vi "SVT Coherent Output Power Subset.vi"(0 "scaled signal X [EUx]":waveform(dbl)={"t0"=timestamp(0 s since 1904-01-01), "dt"=1e-05, "Y"=[]}, 1 "scaled signal Y [EUy]":waveform(dbl)={"t0"=timestamp(0 s since 1904-01-01), "dt"=1e-05, "Y"=[]}, 2 "window":T10=1 items=["None"=0, "Hanning"=1, "Hamming"=2, "Blackman-Harris"=3, "Exact Blackman"=4, "Blackman"=5, "Flat Top"=6, "4 Term B-Harris "=7, "7 Term B-Harris"=8, "Low Sidelobe"=9, "Force - Exponential"=10, "Blackman Nuttall"=11, "Triangle"=30, "Bartlett-Hanning"=31, "Bohman"=32, "Parzen"=33, "Welch"=34, "Kaiser"=60, "Dolph-Chebyshev"=61, "Gaussian"=62], 3 "frequency range":T7={"start frequency"=1000.0, "stop frequency"=5000.0} {"stop frequency" min=0.0 format="%.2f"; "start frequency" min=0.0 format="%.2f"}, 4 "dB On (T)":bool=TRUE, 5 "error in (no error)":errorcluster, 7 "averaging parameters":T8={"averaging mode"=enum."No averaging", "weighting mode"=enum."Exponential", "number of averages"=10, "linear mode"=enum."One shot"}, 8 "force/exp settings":T9={"force window [%]"=50.0, "exp window [%]"=10.0} {"exp window [%]" min=0.0 max=100.0 format="%.2f"; "force window [%]" min=0.0 max=100.0 format="%.2f"}, 9 "restart averaging (F)":bool) -> (11 "averaging done":bool, 12 "coherence":cluster{"f0":dbl, "df":dbl, "coherence":dbl[]}={"f0"=nan, "df"=inf, "coherence"=[]} {"coherence" format="%.2p"; "df" format="%.2p"; "f0" format="%.2p"}, 13 "averages completed":dbl, 14 "coherent output power [dB EUy]":cluster{"f0":dbl, "df":dbl, "magnitude":dbl[]}={"f0"=nan, "df"=inf, "magnitude"=[]} {"magnitude" format="%.2p"; "df" format="%.2p"; "f0" format="%.2p"}, 15 "unit label":string, 18 "spectrum info":T1={"channel name"="", "description"="", "x-axis units"=1, "spectral info"={"spectrum type"=enum."Power [Magnitude^2]", "linear/dB"=enum."linear", "window"=0, "window size"=0, "FFT size"=0}, "engineering units"=0, "custom label"="", "dB reference [EU]"=0.0, "peak units"=enum."rms", "weighting filter"=0, "spectral density?"=FALSE, "unit label"="", "spectrum skewed?"=FALSE, "complimentary spectrum units"=enum."none"} {"x-axis units" items=["Time (s)"=0, "Frequency-CB (Hz)"=1, "Frequency-CPB (Hz)"=1248, "Frequency-Arbitrary (Hz)"=2357, "Quefrency (s)"=2, "Revolutions (rev)"=3, "Order"=4, "Speed (RPM)"=11, "Speed (rad/s)"=21, "Index"=65535]; "weighting filter" items=["Linear", "A-weighting", "B-weighting", "C-weighting", "ITU-R 468-4", "Dolby", "CCITT", "C-message", "Wb", "Wc", "Wd", "We", "Wf", "Wh", "Wj", "Wk", "Wm", "AES17 20 kHz lowpass", "AES17 40 kHz lowpass", "AES17 20 kHz highpass", "AES17 40 kHz highpass"]; "dB reference [EU]" format="%.2f"; "engineering units" items=["custom..."=0, "V"=1, "A"=21, "C"=30, "pC"=31, "s"=32, "-"=29, "Pa"=2, "N"=20, "g"=3, "m/s^2"=4, "m/s"=5, "m"=6, "mm/s"=12, "mm"=13, "micron/s"=14, "micron"=15, "in/s^2"=7, "in/s"=8, "in"=9, "mil/s"=10, "mil"=11, "rad/s^2"=16, "rad/s"=17, "rad"=18, "deg/s^2"=26, "deg/s"=27, "deg"=28, "RPM"=22, "cycle/s^2"=23, "Hz"=24, "cycle"=25, "strain"=19]; "spectral info"."window" items=["None "=0, "Hanning"=1, "Hamming"=2, "Blackman-Harris"=3, "Exact Blackman"=4, "Blackman"=5, "Flat Top"=6, "4 Term B-Harris "=7, "7 Term B-Harris"=8, "Low Sidelobe"=9, "Force - Exponential"=10, "Gaussian"=62]}, 19 "error out":errorcluster)   [LabVIEW 2017]
doc: "Computes a subset of the coherent output power based on <B>scaled signal X [EUx]</B> and <B>scaled signal Y [EUy]</B>. The subset is defined by <B>frequency range</B>."
uses:
  <vilib>/addons/_NISVFA/_Shared subVIs/Controls/svc_Window [Dual FFT].ctl
  <vilib>/addons/_NISVFA/_Shared subVIs/Controls/svc_Spectrum Info.ctl
  <vilib>/addons/_NISVFA/_Shared subVIs/Controls/svc_X-Axis Units.ctl
  <vilib>/addons/_NISVFA/_Shared subVIs/Controls/svc_Spectrum Type.ctl
  <vilib>/addons/_NISVFA/_Shared subVIs/Controls/svc_Engineering Units Text Ring.ctl
  <vilib>/addons/_NISVFA/_Shared subVIs/Controls/svc_Weighting Filter Text Ring.ctl
  <vilib>/addons/_NISVFA/_Shared subVIs/Controls/svc_Complimentary Spectrum Units.ctl
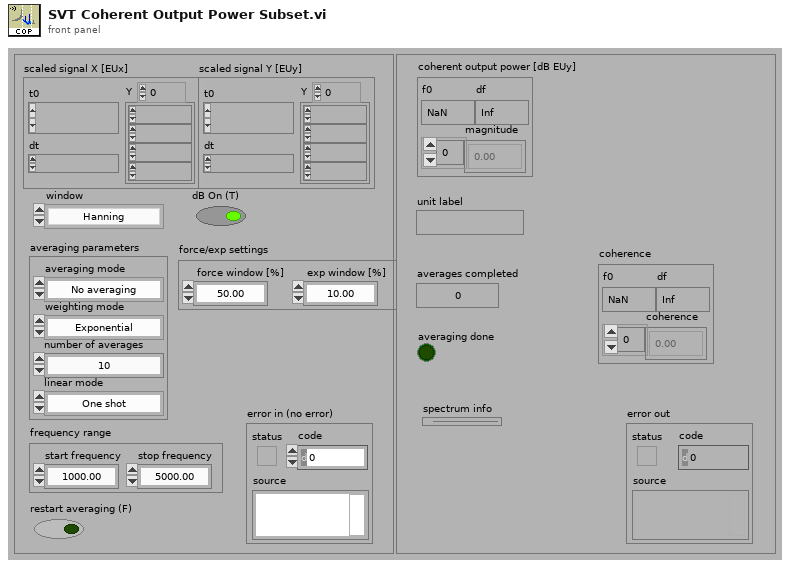
[diagram p1: front panel]
types:
  T1 = typedef "svc_Spectrum Info.ctl" = cluster{"channel name":string, "description":string, "x-axis units":T2, "spectral info":cluster{"spectrum type":T3, "linear/dB":enum16{"linear", "dB"}, "window":u16, "window size":i32, "FFT size":i32}, "engineering units":T4, "custom label":string, "dB reference [EU]":dbl, "peak units":enum16{"rms", "peak", "peak-peak"}, "weighting filter":T5, "spectral density?":bool, "unit label":string, "spectrum skewed?":bool, "complimentary spectrum units":T6}
  T2 = typedef "svc_X-Axis Units.ctl" = u16
  T3 = typedef "svc_Spectrum Type.ctl" = enum16{"FFT Spectrum [complex]", "Amplitude [Magnitude]", "Power [Magnitude^2]", "Cross Spectrum [complex]", "Frequency Response [Complex]"}
  T4 = typedef "svc_Engineering Units Text Ring.ctl" = u16
  T5 = typedef "svc_Weighting Filter Text Ring.ctl" = u16
  T6 = typedef "svc_Complimentary Spectrum Units.ctl" = enum16{"none", "radians", "degrees", "cycles", "imaginary"}
  T7 = cluster{"start frequency":dbl, "stop frequency":dbl}
  T8 = cluster{"averaging mode":enum16{"No averaging", "Vector averaging", "RMS averaging", "Peak hold"}, "weighting mode":enum16{"Linear", "Exponential"}, "number of averages":u32, "linear mode":enum16{"One shot", "Auto restart"}}
  T9 = cluster{"force window [%]":dbl, "exp window [%]":dbl}
  T10 = typedef "svc_Window [Dual FFT].ctl" = u32
  T11 = enum16{"Cross spectrum", "Frequency response", "Coherent output power"}
  T12 = enum16{"Restart processing", "Continue processing", "Skip processing"}
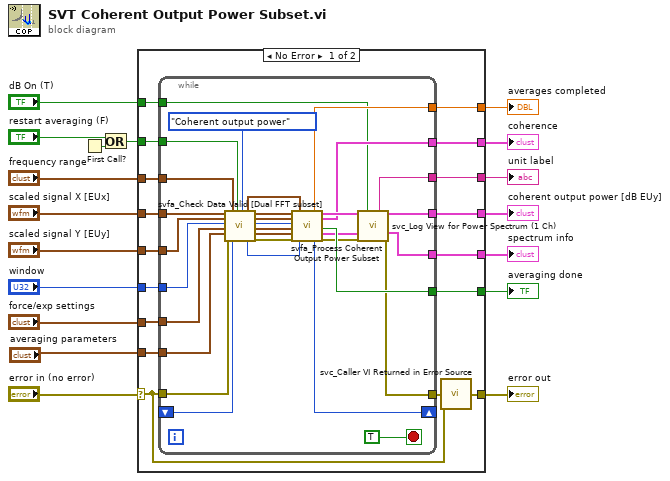
[diagram p0: block diagram]
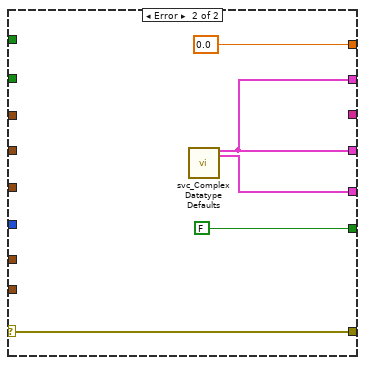
[diagram p2: hidden frame]
diagram:
  n1 = First Call?() -> (First Call?: T/F=w3:bool)
  n2 = Or(x="restart averaging (F)", y=w3) -> (x .or. y?=w1:bool)
  n3 = case shown="No Error" "error in (no error)" {
    selector: "error in (no error)" -> [w19 w71]
    tunnel: "window" -> [w32 _]
    tunnel: "averaging parameters" -> [w34 _]
    tunnel: "dB On (T)" -> [w25 _]
    tunnel: [w20 w71] -> w15
    tunnel: [w23 w68] -> w14
    tunnel: "force/exp settings" -> [w33 _]
    tunnel: "scaled signal X [EUx]" -> [w30 _]
    tunnel: "scaled signal Y [EUy]" -> [w31 _]
    tunnel: w1 -> [w28 _]
    tunnel: [w24 _] -> w9
    tunnel: [w27 0.0 ("averages completed")] -> w8
    tunnel: [w35 FALSE ("averaging done")] -> w7
    tunnel: "frequency range" -> [w29 _]
    tunnel: [w26 w68] -> w5
    tunnel: [w21 w67] -> w4
    frame No Error {
      n4 = while {
        tunnel: [w39] -> w21
        tunnel: [w38] -> w22
        tunnel: [w40] -> w23
        tunnel: [w41] -> w24
        tunnel: w25 -> [w42]
        tunnel: [w43] -> w26
        tunnel: [w56] -> w27
        shift-left: _ -> [w57]
        shift-right: [w46] -> _
        tunnel: w28 -> [w59]
        tunnel: w29 -> [w60]
        tunnel: w30 -> [w61]
        tunnel: w31 -> [w62]
        tunnel: w32 -> [w63]
        tunnel: w33 -> [w64]
        tunnel: w34 -> [w65]
        tunnel: w19 -> [w66]
        tunnel: [w55] -> w35
        stop <- TRUE stop-if-true
        n5 = call <vilib>:"svfa_Check Data Valid [Dual FFT subset].vi"("stimulus [X]"=w61, "response [Y]"=w62, "window"=w63, "force/exp settings"=w64, "averaging parameters"=w65, "error in (no error)"=w66, "frequency range"=w60, "processing control in"=w57, "restart averaging (F)"=w59, "measurement"=T11."Coherent output power") -> ("dup frequency range"=w54:T7, "processing control out"=w47:T12, "dup stimulus [X]"=w53:waveform(dbl), "dup response [Y]"=w52:waveform(dbl), "window"=w51:u16, "dup force/exp settings"=w50:T9, "dup averaging parameters"=w49:T8, "error out"=w48:errorcluster)  [unwired: 1 in, 1 out]
        n6 = call <vilib>:"svfa_Process Coherent Output Power Subset.vi"("Windowed signal [X]"=w53, "Windowed signal [Y]"=w52, "window"=w51, "force/exp settings"=w50, "averaging parameters"=w49, "error in (no error)"=w48, "Spectrum Settings"=w54, "processing control"=w47) -> ("averages completed"=w56:dbl, "processing control"=w46:T12, "COP"=w45:cluster{"df":dbl, "df":dbl, dbl[]}, "coherence"=w43:cluster{"f0":dbl, "df":dbl, "coherence":dbl[]}, "averaging done"=w55:bool, "spectrum info"=w44:T1, "error out"=w36:errorcluster)  [unwired: 5 in]
        n7 = call <vilib>:"svc_Log View for Power Spectrum (1 Ch).vi"("power spectrum [dB EU]"=w45, "dB On (T)"=w42, "spectrum info"=w44, "error in (no error)"=w36) -> ("unit label"=w41:string, "power spectrum [dB EU]"=w40:cluster{"f0":dbl, "df":dbl, "magnitude":dbl[]}, "spectrum info out"=w39:T1, "error out"=w38:errorcluster)  [unwired: 8 in]
      }
      n8 = call <vilib>:"svc_Caller VI Returned in Error Source.vi"("warning input to caller"=w19, "error in (no error)"=w22) -> ("error out"=w20:errorcluster)  [unwired: 3 in]
    }
    frame Error {
      n9 = call <vilib>:"svc_Complex Datatype Defaults.vi"() -> ("empty spectrum"=w68:cluster{"f0":dbl, "df":dbl, "magnitude":dbl[]}, "dead spectrum info"=w67:T1)  [unwired: 11 in, 7 out]
    }
  }
  "error out" <- w15
  "coherent output power [dB EUy]" <- w14
  "unit label" <- w9
  "averages completed" <- w8
  "averaging done" <- w7
  "spectrum info" <- w4
  "coherence" <- w5
